vi "Main Page.vi"(8 "error in":errorcluster, 11 "Node Ptr":T1 format="%.0x") -> (0 "error out":errorcluster)   [LabVIEW 2020, in "AIM ARINC 429 System Explorer.lvlib" / "Implementation.lvlib"]
uses:
  Implementation.lvlib
  <vilib>/NI VeriStand/Custom Device API/Custom Device API.lvlib
  Scripting/AIM/AIM ARINC 429 Scripting.lvlib
  Scripting/AIM/Constants.vi
  <vilib>/NI VeriStand/Custom Device API/Custom Device Item Ref.ctl
panel:
  in  "General Header":cluster{"Section Name":string}={"Section Name"="Ballard ARINC 429 - Main"}
  in  "Number":u8=1 caption="PXI Slot Number"
  in  "SHDocVw.IWebBrowser":refnum<k7>(container)
  in  "Description":string
  in  "Name":string
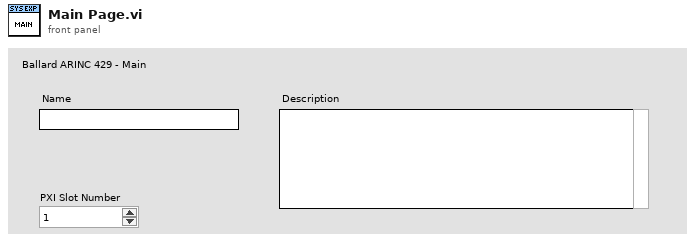
[diagram p1: front panel]
types:
  T1 = typedef "Custom Device API.lvlib/Custom Device Item Ref.ctl" = u64
  T2 = typedef "Device Parameters.ctl" = cluster{"pxi slot":u8}
  T3 = typedef "Custom Device API.lvlib/Custom Device Item Info.ctl" = cluster{"Name":string, "Is Channel":bool, "GUID":string, "Is Waveform":bool}
  T4 = typedef "Custom Device API.lvlib/Custom Device Commands.ctl" = enum16{"Default", "Item renamed", "Shutdown", "Dynamic button pressed"}
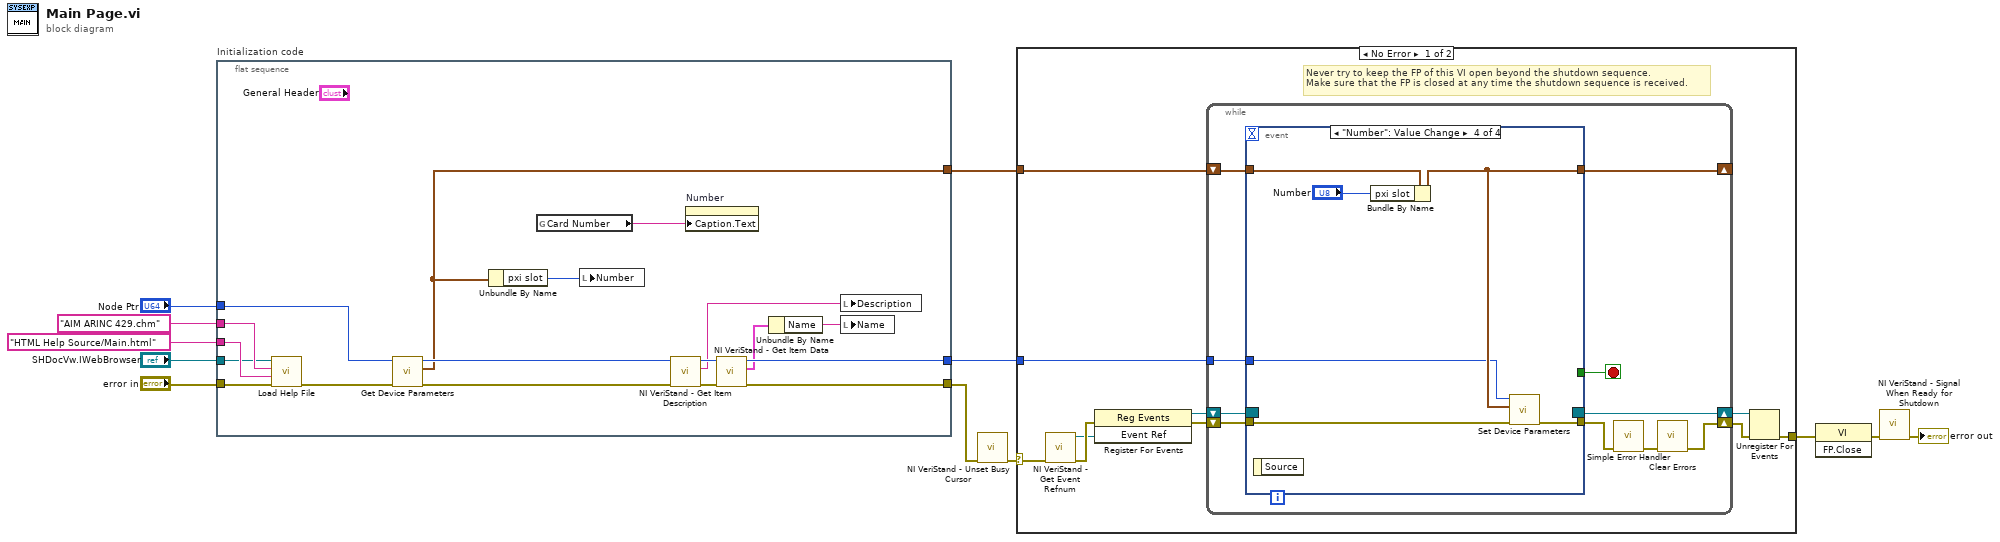
[diagram p0: block diagram]
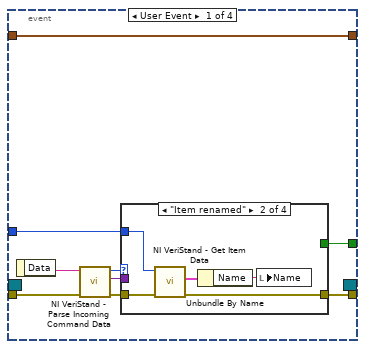
[diagram p2: hidden frame]
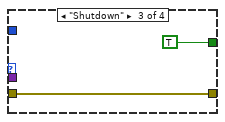
[diagram p4: hidden frame]
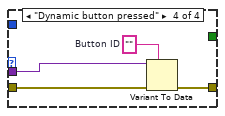
[diagram p5: hidden frame]
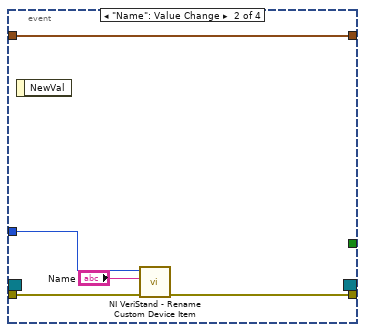
[diagram p6: hidden frame]
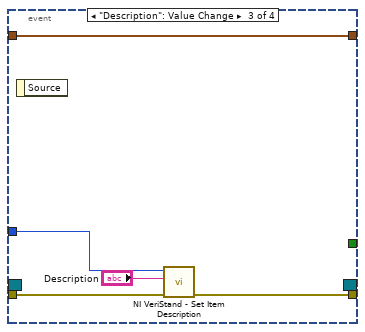
[diagram p7: hidden frame]
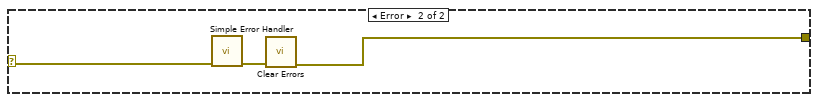
[diagram p8: hidden frame]
diagram:
  n1 = flat-sequence "Initialization code" {
    tunnel: "error in" -> [w23]
    tunnel: "Node Ptr" -> [w16]
    tunnel: [w26] -> w8
    tunnel: [w30] -> w5
    tunnel: "SHDocVw.IWebBrowser" -> [w20]
    tunnel: "HTML Help Source/Main.html" ("HTML File") -> [w21]
    tunnel: "AIM ARINC 429.chm" ("CD_CHM_FileName") -> [w22]
    tunnel: [w15] -> w1
    frame #0 {
      n2 = call "Load Help File.vi"("error in (no error)"=w23, "HTML File to Load"=w21, "Main CHM File"=w22, "Browser"=w20) -> ("error out"=w19:errorcluster)  [unwired: 7 in]
      n3 = call "Get Device Parameters.vi"("error in"=w19, "AIM ARINC 429 custom device in"=w16) -> ("error out"=w18:errorcluster, "device parameters"=w15:T2, "AIM ARINC 429 custom device out"=w17:T1)  [unwired: 7 in]
      n4 = Unbundle By Name(w15) -> ("pxi slot"=w13:u8)
      n5 = global read "Constants.vi" "Card Number"() -> (w14:string)
      n6 = local write "Number"(w13) -> ()
      n7 = call <vilib>:"NI VeriStand - Get Item Description.vi"("error in (no error)"=w18, "Item Ref in"=w17) -> ("error out"=w28:errorcluster, "Description"=w24:string, "Item Ref out"=w29:T1)  [unwired: 7 out]
      n8 = property on="Number" class="DigNum (strict)"("Caption.Text"=w14) -> ()  [unwired: 2 in, 2 out]
      n9 = call <vilib>:"NI VeriStand - Get Item Data.vi"("error in (no error)"=w28, "Item Ref in"=w29) -> ("error out"=w26:errorcluster, "Item Info"=w27:T3, "Item Ref out"=w30:T1)  [unwired: 7 out]
      n10 = Unbundle By Name(w27) -> ("Name"=w25:string)
      n11 = local write "Description"(w24) -> ()
      n12 = local write "Name"(w25) -> ()
    }
  }
  n13 = call <vilib>:"NI VeriStand - Unset Busy Cursor.vi"("error in (no error)"=w8) -> ("error out"=w7:errorcluster)  [unwired: 10 out]
  n14 = case shown="No Error" w7 {
    selector: w7 -> [w32 w90]
    tunnel: [w37 w88] -> w12
    tunnel: w5 -> [w33 _]
    tunnel: w1 -> [w31 _]
    frame No Error {
      # "Never try to keep the FP of this VI open beyond the shutdown sequence.\nMake sure that the FP is closed at any time the shutdown sequence is received."
      n15 = call <vilib>:"NI VeriStand - Get Event Refnum.vi"("error in (no error)"=w32) -> ("error out"=w40:errorcluster, "Event Ref"=w36:refnum<user-event>)  [unwired: 9 out]
      n16 = register-events(error in=w40, w36) -> (reference out=w34:refnum<event-registration>, error out=w35:errorcluster)  [unwired: 1 in]
      n17 = while {
        tunnel: w33 -> [w46]
        shift-right: [w43] -> w38
        shift-left: w35 -> [w49]
        shift-right: [w50] -> w39
        shift-left: w34 -> [w48]
        shift-right: [w41] -> _
        shift-left: w31 -> [w42]
        stop <- w47 stop-if-true
        n18 = event shown="[3] \"Number\": Value Change" {
          selector: w48 -> [_ _ _ _]
          dyn-events: [_ _ _ _] -> w50
          timeout: _ -> [_ _ _ _]
          tunnel: w49 -> [w59 w76 w80 w85]
          tunnel: [w55 _ _ _] -> w47
          tunnel: [w54 w75 w79 w84] -> w45
          tunnel: w46 -> [w53 w74 w81 w82]
          tunnel: w42 -> [w51 w72 w77 w87]
          tunnel: [w51 w72 w77 w86] -> w41
          event User Event {
            n19 = event-data() -> ("Data"=w58:string)  [unwired: 1 out]
            n20 = call <vilib>:"NI VeriStand - Parse Incoming Command Data.vi"("error in (no error)"=w59, "Incoming data"=w58) -> ("error out"=w57:errorcluster, "Outgoing data"=w52:variant, "Action"=w56:T4)  [unwired: 7 out]
            n21 = case shown="\"Item renamed\"" w56 {
              tunnel: w57 -> [w60 w65 w66 w71]
              tunnel: [_ _ TRUE _] -> w55
              tunnel: [w60 w62 w66 w68] -> w54
              tunnel: w53 -> [_ w64 _ _]
              tunnel: w52 -> [_ _ _ w70]
              frame "Default", Default {
              }
              frame "Item renamed" {
                n22 = call <vilib>:"NI VeriStand - Get Item Data.vi"("error in (no error)"=w65, "Item Ref in"=w64) -> ("error out"=w62:errorcluster, "Item Info"=w63:T3)  [unwired: 8 out]
                n23 = Unbundle By Name(w63) -> ("Name"=w61:string)
                n24 = local write "Name"(w61) -> ()
              }
              frame "Shutdown" {
              }
              frame "Dynamic button pressed" {
                w69 = ""  # Button ID
                n25 = Variant To Data(error in=w71, type=w69, Variant=w70) -> (error out=w68:errorcluster)  [unwired: 1 out]
              }
            }
          }
          event "Name": Value Change {
            n26 = event-data() -> ()  [unwired: 2 out]
            n27 = call <vilib>:"NI VeriStand - Rename Custom Device Item.vi"("error in (no error)"=w76, "New Name"="Name", "Item Ref in"=w74) -> ("error out"=w75:errorcluster)  [unwired: 1 in, 7 out]
          }
          event "Description": Value Change {
            n28 = event-data() -> ()  [unwired: 2 out]
            n29 = call <vilib>:"NI VeriStand - Set Item Description.vi"("error in (no error)"=w80, "Description"="Description", "Item Ref in"=w81) -> ("error out"=w79:errorcluster)  [unwired: 8 out]
          }
          event "Number": Value Change {
            n30 = event-data() -> ()  [unwired: 2 out]
            n31 = Bundle By Name(cluster=w87, "pxi slot"="Number") -> (w86:T2)
            n32 = call "Set Device Parameters.vi"("error in"=w85, "device parameters"=w86, "AIM ARINC 429 custom device in"=w82) -> ("error out"=w84:errorcluster)  [unwired: 7 in, 1 out]
          }
        }
        n33 = call <vilib>:"Simple Error Handler.vi"("error in (no error)"=w45) -> ("error out"=w44:errorcluster)  [unwired: 1 in, 7 out]
        n34 = call <vilib>:"Clear Errors.vi"("error in (no error)"=w44) -> ("error out"=w43:errorcluster)  [unwired: 1 in, 5 out]
      }
      n35 = Unregister For Events(event registration refnum=w39, error in=w38) -> (error out=w37:errorcluster)
    }
    frame Error {
      n36 = call <vilib>:"Simple Error Handler.vi"("error in (no error)"=w90) -> ("error out"=w89:errorcluster)  [unwired: 1 in, 7 out]
      n37 = call <vilib>:"Clear Errors.vi"("error in (no error)"=w89) -> ("error out"=w88:errorcluster)  [unwired: 1 in, 5 out]
    }
  }
  n38 = invoke class="VI" method="FP.Close"(error in=w12) -> (error out=w11:errorcluster)  [unwired: 2 in, 2 out]
  n39 = call <vilib>:"NI VeriStand - Signal When Ready for Shutdown.vi"("error in (no error)"=w11) -> ("error out"=→"error out":errorcluster)  [unwired: 10 out]
